vi "Finalize Interpreter.vi"(8 "error in (no error)":errorcluster) -> (0 "error out":errorcluster)   [LabVIEW 2020, in "G-Embedded-Python-Interpreter-Toolkit.lvlib"]
uses:
  G-Embedded-Python-Interpreter-Toolkit.lvlib
  bin/gepit.cp310.32.dll
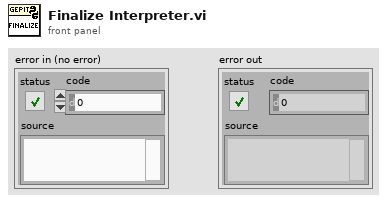
[diagram p1: front panel]
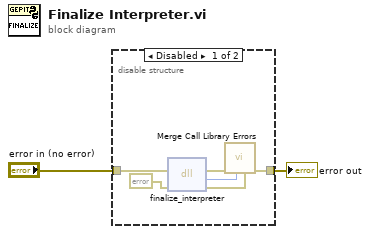
[diagram p0: block diagram]
diagram:
  n1 = disable-structure shown="Disabled" {
    disable-tunnel: "error in (no error)" -> [w7 w9]
    disable-tunnel: [w6 w9] -> w1
    frame Disabled {
      n2 = dll-call lib="C:/serenial/libraries/g-embedded-python-interpreter-toolkit/LabVIEW/bin/gepit.cp310.32.dll" fn="finalize_interpreter"(error in=w7, "Error"=errorcluster {"status"=FALSE, "code"=0, "source"=""} ("error constant")) -> (error out=w5:errorcluster, "return type"=w4:i32, "Error"=w3:errorcluster)  [unwired: 2 in, 1 out]
      n3 = call "Merge Call Library Errors.vi"("Call Library Error"=w3, "Return Value"=w4, "error in"=w5) -> ("error out"=w6:errorcluster)  [unwired: 8 in]
    }
    frame Enabled {
      # "Probably Safer to Just Leave the Interpreter Going"
    }
  }
  "error out" <- w1
